vi "0-Rotate Boat Overlays.vi"(4 "Overlay References In":T1) -> (1 "Rotated Boat Icon Bitmap Out":u32[][](array[colorbox]), 2 "Boat Icon Out":T2(plugin-control))   [LabVIEW 2011]
doc: "Rotates icon images of the boat and sails and overlays them on each other to create a representation of the current state of the robot. Also converts the output image to a bitmap for easy overlay on the mission map.\n\nby Jason Curtis"
uses:
  2-Think/2 Typedefs/heading.ctl
  2-Think/2 Typedefs/sail setpt.ctl
  0 Typedefs/Overlay References.ctl
  <vilib>/vision/Image Controls.llb/IMAQ Image.ctl
  2-Think/2 Globals/2 Global.vi
  <vilib>/vision/NI_Vision_Development_Module.lvlib
panel:
  out "Sail Position":T3
  out "Heading":T4 format="%05.1f"
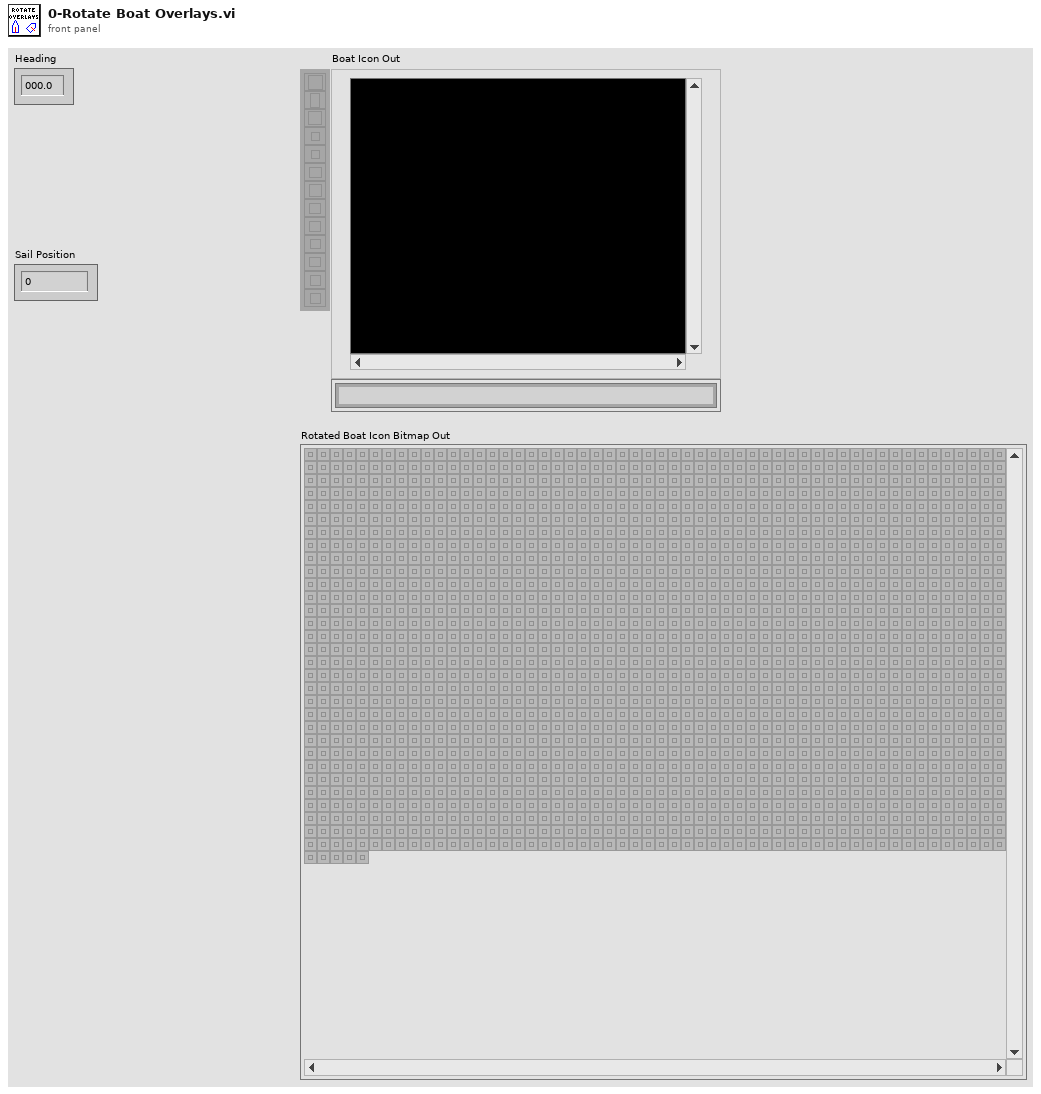
[diagram p1: front panel]
types:
  T1 = typedef "Overlay References.ctl" = cluster{"Boat Icon, Unroatated":T2, "Boat Icon, Rotated":T2, "Sail Icon, Unrotated":T2, "Sail Icon, Rotated":T2}
  T2 = typedef "IMAQ Image.ctl" = refnum<image>
  T3 = typedef "sail setpt.ctl" = dbl
  T4 = typedef "heading.ctl" = dbl
  T5 = typedef "setpoints to boat.ctl" = cluster{"Sail Position":T3, "Rudder Angle":T6}
  T6 = typedef "rudder angle.ctl" = dbl
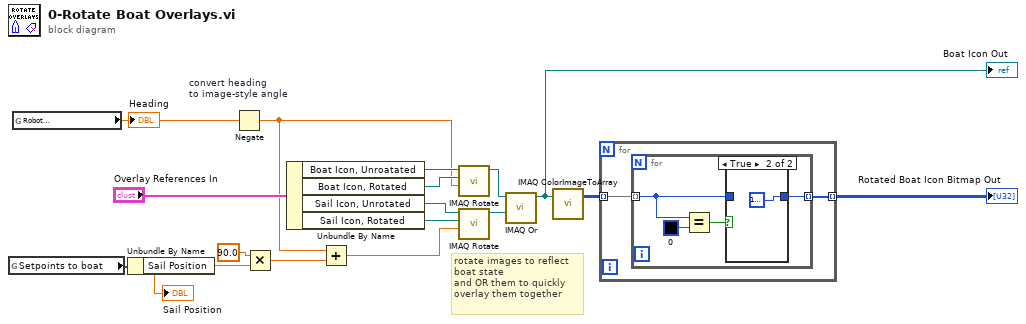
[diagram p0: block diagram]
diagram:
  # "rotate images to reflect\nboat state\nand OR them to quickly \noverlay them together"
  n1 = global read "2 Global.vi" "Setpoints to boat"() -> (w3:T5)
  n2 = global read "2 Global.vi" "Robot\nHeading"() -> (w1:T4)
  "Heading" <- w1
  n3 = Unbundle By Name(w3) -> ("Sail Position"=w2:T3)
  "Sail Position" <- w2
  n4 = Negate "convert heading\nto image-style angle"(x=w1) -> (-x=w4:T4)
  n5 = Multiply(x=T4 90.0 ("Heading 2"), y=w2) -> (x*y=w5:T4)
  n6 = Unbundle By Name("Overlay References In") -> ("Boat Icon, Unroatated"=w17:T2, "Boat Icon, Rotated"=w16:T2, "Sail Icon, Unrotated"=w14:T2, "Sail Icon, Rotated"=w15:T2)
  n7 = Add(x=w4, y=w5) -> (x+y=w7:T4)
  n8 = call "IMAQ Rotate"("Angle (degrees)"=w4, "Image Dst"=w16, "Image Src"=w17) -> ("Image Dst Out"=w10:T2)  [unwired: 7 in, 1 out]
  n9 = call "IMAQ Rotate"("Angle (degrees)"=w7, "Image Dst"=w15, "Image Src"=w14) -> ("Image Dst Out"=w11:T2)  [unwired: 7 in, 1 out]
  n10 = call "IMAQ Or"("Image Src B"=w11, "Image Src A"=w10) -> ("Image Dst Out"=w12:T2)  [unwired: 8 in, 1 out]
  "Boat Icon Out" <- w12
  n11 = call "IMAQ ColorImageToArray"("Image"=w12) -> ("Image Pixels (U32)"=w8:u32[][])  [unwired: 2 in, 3 out]
  n12 = for {
    tunnel: w8 -> [w19] mode=indexing
    tunnel: [w18] -> w9 mode=indexing
    n13 = for {
      tunnel: w19 -> [w21] mode=indexing
      tunnel: [w22] -> w18 mode=indexing
      n14 = Equal?(x=w21, y=u32 0) -> (x = y?=w23:bool)
      n15 = case shown="True" w23 {
        tunnel: [w24 u32 16777216] -> w22
        tunnel: w21 -> [w24 _]
        frame False {
        }
        frame True {
        }
      }
    }
  }
  "Rotated Boat Icon Bitmap Out" <- w9
